vi "Test merging in FPGA.vi"() -> ()   [LabVIEW 2019]
panel:
  out "Array 2":u32[][](array[colorbox])
  out "Array":u32[](array[numeric])
  out "Numeric":i32
  out "Row index":u32
  in  "Row":i16
  in  "Col":i16
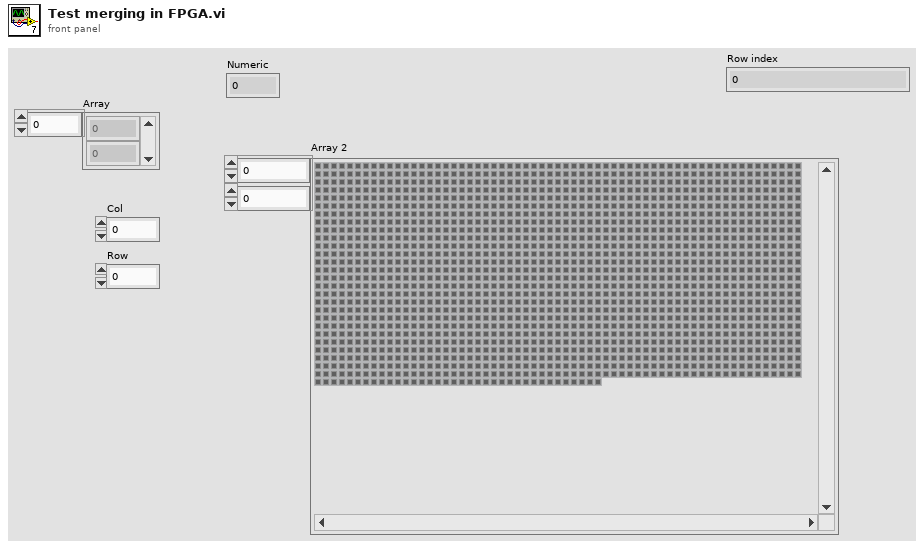
[diagram p1: front panel]
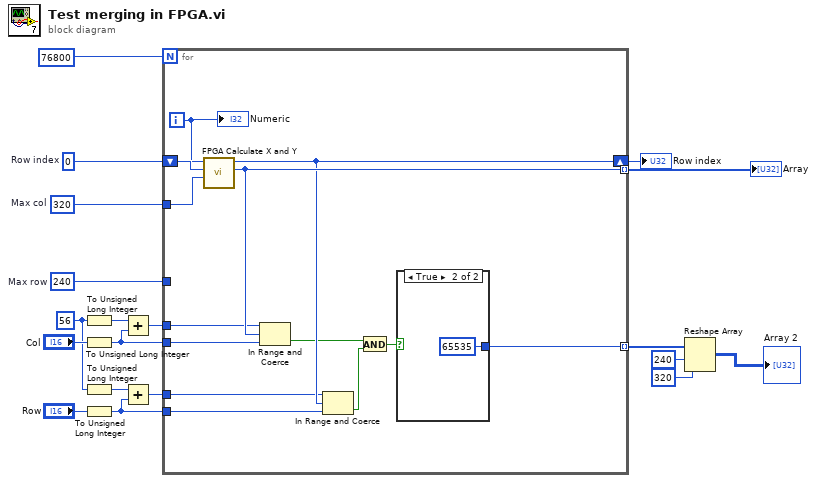
[diagram p0: block diagram]
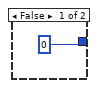
[diagram p2: hidden frame]
diagram:
  w16 = u32 0  # Row index
  w17 = i16 240  # Max row
  w18 = i16 320  # Max col
  w6 = i16 56
  n1 = To Unsigned Long Integer(number=w6) -> (unsigned 32bit integer=w10:u32)
  n2 = To Unsigned Long Integer(number="Col") -> (unsigned 32bit integer=w11:u32)
  n3 = To Unsigned Long Integer(number=w6) -> (unsigned 32bit integer=w9:u32)
  n4 = To Unsigned Long Integer(number="Row") -> (unsigned 32bit integer=w7:u32)
  n5 = Add(x=w10, y=w11) -> (x+y=w12:u32)
  n6 = Add(x=w9, y=w7) -> (x+y=w5:u32)
  n7 = for {
    N: 76800 -> [_]
    tunnel: w11 -> [w27]
    tunnel: w18 -> [w30]
    tunnel: w17 -> [_]
    shift-right: [w26] -> w15
    shift-left: w16 -> [w32]
    tunnel: [w29] -> w14 mode=indexing
    tunnel: w12 -> [w28]
    tunnel: w7 -> [w24]
    tunnel: w5 -> [w25]
    tunnel: [w20] -> w4 mode=indexing
    i -> [w31]
    n8 = call "FPGA Calculate X and Y.vi"("Max col"=w30, "Row index in"=w32, "Current Interation"=w31) -> ("Col index out"=w29:u32, "Row index out"=w26:u32)  [unwired: 7 in]
    n9 = In Range and Coerce(upper limit=w28, x=w29, lower limit=w27) -> (In Range?=w22:bool)  [unwired: 1 out]
    n10 = In Range and Coerce(upper limit=w25, x=w26, lower limit=w24) -> (In Range?=w23:bool)  [unwired: 1 out]
    n11 = And(x=w22, y=w23) -> (x .and. y?=w21:bool)
    n12 = case shown="True" w21 {
      tunnel: [0 65535] -> w20
      frame False {
      }
      frame True {
      }
    }
    "Numeric" <- w31
  }
  "Row index" <- w15
  "Array" <- w14
  n13 = Reshape Array(w4, 240 ("dimension size"), 320 ("dimension size")) -> (→"Array 2":i32[][])
